vi "Test.vi"() -> ()   [LabVIEW 2016]
uses:
  PCANUSB.lvclass
  PCAN/CAN Communication.llb/CAN MSG Cluster.ctl
  PCAN/CAN Communication.llb/TPCANBaudrate.ctl
panel:
  in  "Boolean":bool
  out "Data":u8[](array[numeric]) format="%x"
  out "CAN_Message out":T1 {"MSG type" format="%x"; "ID" format="%.0x"}
  in  "stop":bool
  in  "error in (no error)":errorcluster
  in  "PCANUSB in":refnum<class "PCANUSB.lvclass">
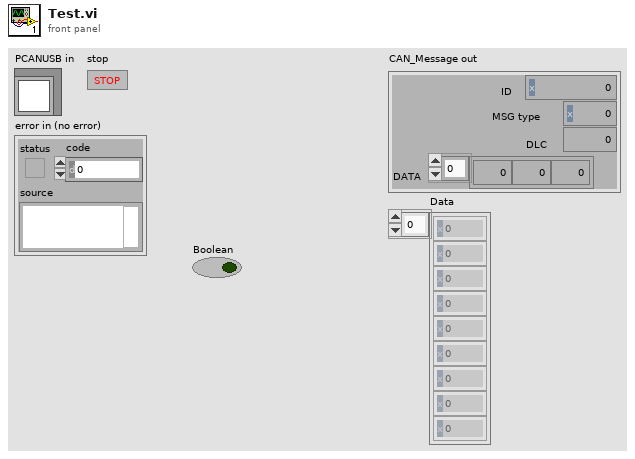
[diagram p1: front panel]
types:
  T1 = typedef "CAN MSG Cluster.ctl" = cluster{"ID":u32, "MSG type":u8, "DLC":u8, "DATA":u8[]}
  T2 = typedef "TPCANBaudrate.ctl" = enum16{"PCAN_BAUD_1M 0x0014", "PCAN_BAUD_800K 0x0016", "PCAN_BAUD_500K 0x001C", "PCAN_BAUD_250K 0x011C", "PCAN_BAUD_125K 0x031C", "PCAN_BAUD_100K 0x432F", "PCAN_BAUD_95K 0xC34E", "PCAN_BAUD_83K 0x852B", "PCAN_BAUD_50K 0x472F", "PCAN_BAUD_47K 0x1414", "PCAN_BAUD_33K 0x8B2F", "PCAN_BAUD_20K 0x532F", "PCAN_BAUD_10K 0x672F", "PCAN_BAUD_5K 0x7F7F", "User Baudrate"}
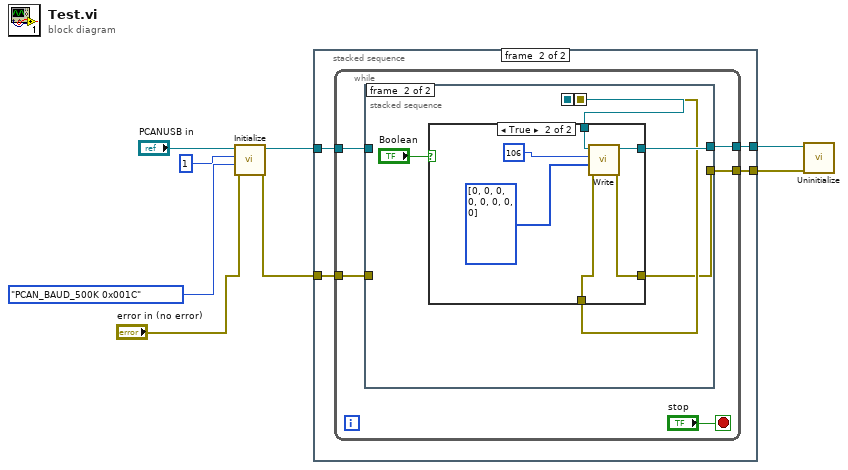
[diagram p0: block diagram]
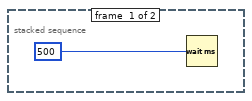
[diagram p2: hidden frame]
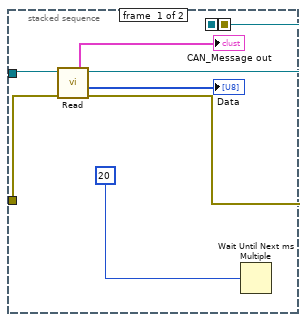
[diagram p3: hidden frame]
diagram:
  n1 = call "Initialize.vi"("error in (no error)"="error in (no error)", "TPCANBaudrate"=TPCANBaudrate."PCAN_BAUD_500K 0x001C", "Channel(1~6)"=u8 1 ("Channel"), "PCANUSB in"="PCANUSB in") -> ("error out"=w4:errorcluster, "PCANUSB out"=w5:refnum<class "PCANUSB.lvclass">)  [unwired: 6 in]
  n2 = stacked-sequence {
    tunnel: w5 -> [_ w13]
    tunnel: w4 -> [_ w12]
    tunnel: [_ w11] -> w3
    tunnel: [_ w10] -> w2
    frame #0 {
      n3 = Wait (ms)(milliseconds to wait=u32 500) -> ()  [unwired: 1 out]
    }
    frame #1 {
      n4 = while {
        tunnel: w13 -> [w17]
        tunnel: w12 -> [w16]
        tunnel: [w15] -> w11
        tunnel: [w14] -> w10
        stop <- "stop" stop-if-true
        n5 = stacked-sequence {
          seq-local: [w20 _] -> [_ w30]
          seq-local: [w19 _] -> [_ w28]
          tunnel: w17 -> [w25 _]
          tunnel: w16 -> [w24 _]
          tunnel: [_ w29] -> w15
          tunnel: [_ w27] -> w14
          frame #0 {
            n6 = call "Read.vi"("error in (no error)"=w24, "PCANUSB in"=w25) -> ("error out"=w19:errorcluster, "Data"=→"Data":u8[], "PCANUSB out"=w20:refnum<class "PCANUSB.lvclass">, "CAN_Message out"=→"CAN_Message out":T1)  [unwired: 4 in, 2 out]
            n7 = Wait Until Next ms Multiple(millisecond multiple=u32 20) -> ()  [unwired: 1 out]
          }
          frame #1 {
            n8 = case shown="True" "Boolean" {
              tunnel: w30 -> [w32 w38]
              tunnel: [w32 w37] -> w29
              tunnel: w28 -> [w31 w36]
              tunnel: [w31 w35] -> w27
              frame False {
              }
              frame True {
                n9 = call "Write.vi"("error in (no error)"=w36, "Data"=u8[] [0, 0, 0, 0, 0, 0, 0, 0], "ID"=u32 106, "PCANUSB in"=w38) -> ("error out"=w35:errorcluster, "PCANUSB out"=w37:refnum<class "PCANUSB.lvclass">)  [unwired: 6 in]
              }
            }
          }
        }
      }
    }
  }
  n10 = call "Uninitialize.vi"("error in (no error)"=w2, "PCANUSB in"=w3) -> ()  [unwired: 8 in, 2 out]
